vi "Tortoisegit commit.vi"(8 "error in (no error)":errorcluster, 10 "path":path, 11 "TortoiseGitProc.exe":path) -> (0 "error out":errorcluster)   [LabVIEW 2017]
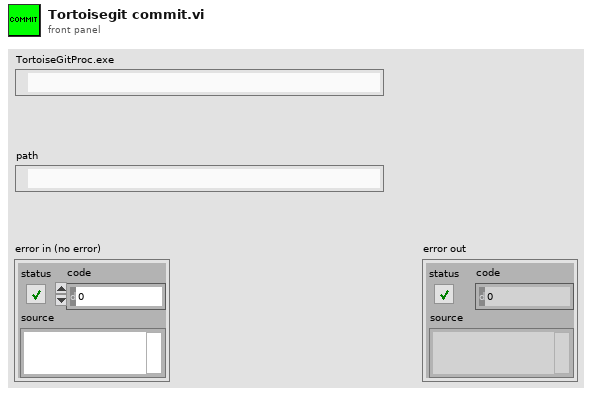
[diagram p1: front panel]
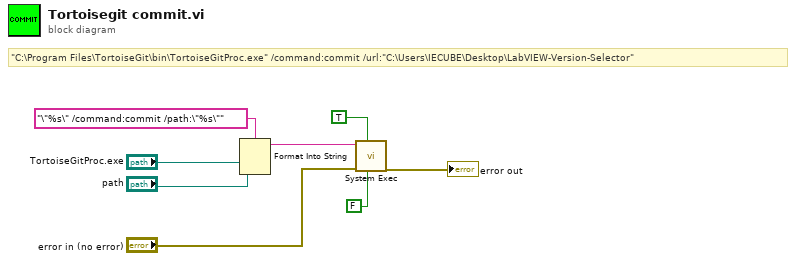
[diagram p0: block diagram]
diagram:
  # "\"C:\\Program Files\\TortoiseGit\\bin\\TortoiseGitProc.exe\" /command:commit /url:\"C:\\Users\\IECUBE\\Desktop\\LabVIEW-Version-Selector\""
  n1 = Format Into String(format string="\"%s\" /command:commit /path:\"%s\"", "TortoiseGitProc.exe", "path") -> (resulting string=w1:string)  [unwired: 2 in, 1 out]
  n2 = call <vilib>:"System Exec.vi"("run minimized? (F)"=FALSE, "wait until completion? (T)"=TRUE, "error in (no error)"="error in (no error)", "command line"=w1) -> ("error out"=→"error out":errorcluster)  [unwired: 4 in, 3 out]
